vi "SimpleShiftRegister.vi"(6 "Limit":i32, 8 "Shift register boolean input":bool, 9 "Shift register integer input":i32) -> (0 "x = y?":bool, 2 "Shift register boolean output":bool, 3 "Shift register integer output":i32)   [LabVIEW 2020, in "WritingDataFile.lvlib"]
uses:
  WritingDataFile.lvlib
panel:
  out "Counter":i32
  in  "stop":bool
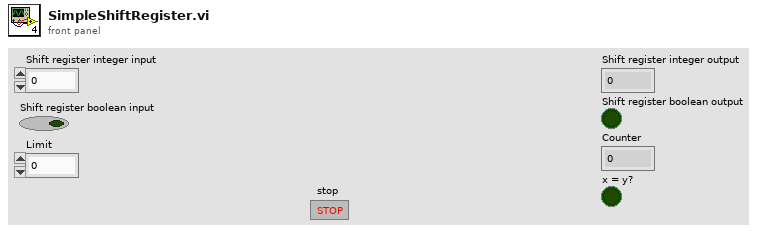
[diagram p1: front panel]
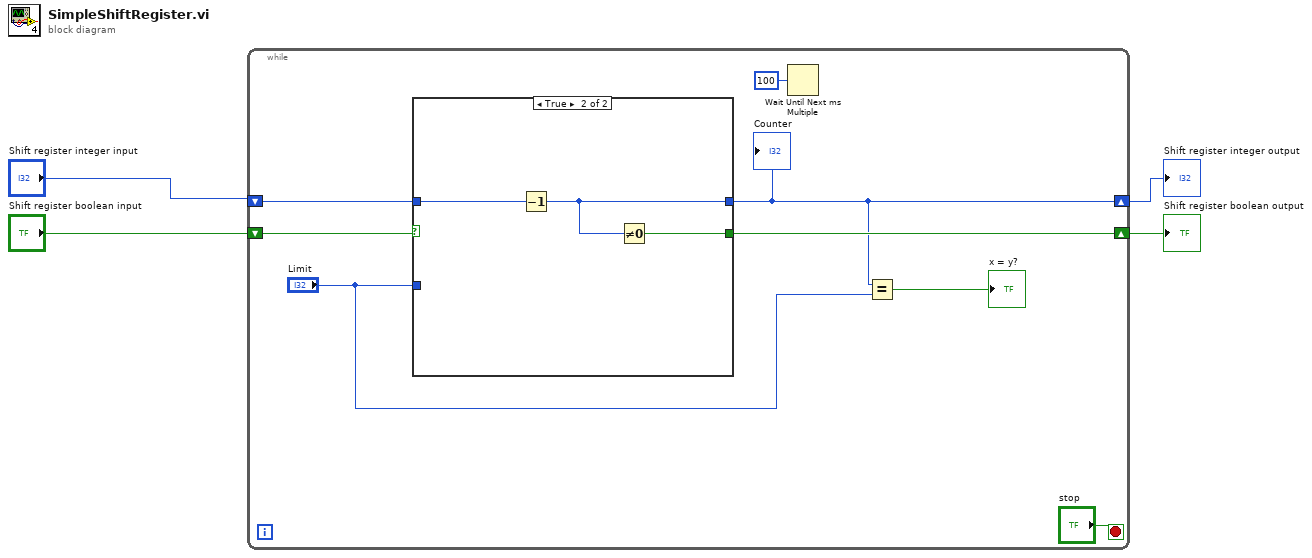
[diagram p0: block diagram]
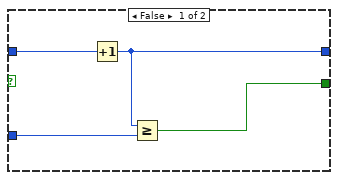
[diagram p2: hidden frame]
diagram:
  n1 = while {
    shift-right: [w7] -> w2
    shift-left: "Shift register integer input" -> [w11]
    shift-right: [w9] -> w1
    shift-left: "Shift register boolean input" -> [w10]
    stop <- "stop" stop-if-true
    n2 = case shown="True" w10 {
      tunnel: [w14 w17] -> w7
      tunnel: w11 -> [w16 w19]
      tunnel: "Limit" -> [w15 _]
      tunnel: [w13 w18] -> w9
      frame False {
        n3 = Increment(x=w16) -> (x+1=w14:i32)
        n4 = Greater Or Equal?(x=w14, y=w15) -> (x >= y?=w13:bool)
      }
      frame True {
        n5 = Decrement(x=w19) -> (x-1=w17:i32)
        n6 = Not Equal To 0?(x=w17) -> (x != 0?=w18:bool)
      }
    }
    "Counter" <- w7
    n7 = Wait Until Next ms Multiple(millisecond multiple=u32 100) -> ()  [unwired: 1 out]
    n8 = Equal?(x=w7, y="Limit") -> (x = y?=→"x = y?":bool)
  }
  "Shift register integer output" <- w2
  "Shift register boolean output" <- w1
